vi "Initialize Battle Dialog.vi"() -> (1 "# Players":i32, 2 "Dashboard":T1[](array[typedef]), 3 "SquareBattle out":refnum<class "SquareBattle.lvclass">, 4 "Intensity Graph Values":cluster{dbl, u32}[](array[cluster]), 6 "Continue?":bool)   [LabVIEW 2014, in "SquareBattle.lvclass"]
uses:
  SquareBattle.lvclass
  Dashboard.ctl
  Runner/Runner.lvclass
  Runner/Runner.lvclass/Runner.ctl
  Runner Cluster.ctl
  SquareBattle.lvclass/SquareBattle.ctl
  Endigit Library/Endigit.lvlib
panel:
  in  "Default Colors":u32[](array[colorbox])=[11163013, 4877194, 13936746, 10864227, 9567230, 16776960, 12868095, 16762130]
  in  "Background Color":u32(colorbox)
  in  "Players":cluster{"Player":u16, "Color":u32}[](array[cluster]) {"Player" items=["Sleepy Engineer"=2, "Sleepy Engineer"=3, "Sleepy Engineer"=4, "Sleepy Engineer"=5, "Shawn the Explorer"=6, "Robert"=8, "Shawn the Wanderer"=9]}
  in  "Cancel":bool
  in  "Start":bool
  in  "Board size":i32=150
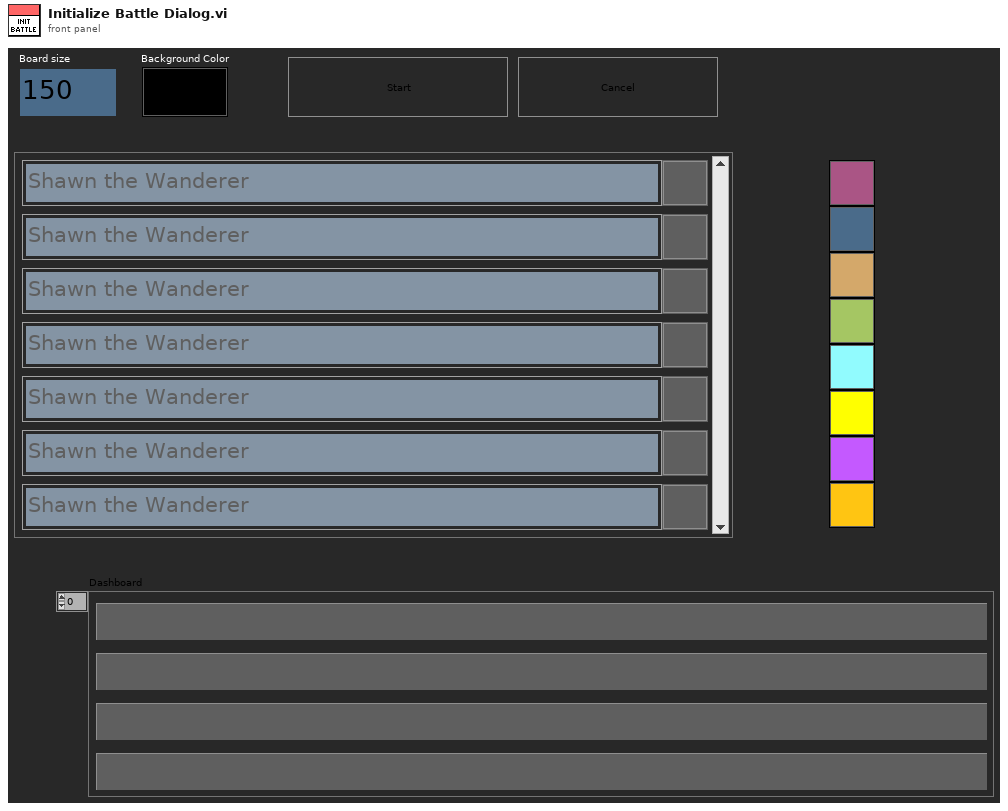
[diagram p1: front panel]
types:
  T1 = typedef "SquareBattle.lvclass/Dashboard.ctl" = cluster{"Color":u32, "Player":string, "Status":string}
  T2 = typedef "SquareBattle.lvclass/Player Info.ctl" = cluster{"Name":string, "Color Box":u32, "Gloat Phrase":string}
  T3 = typedef "SquareBattle.lvclass/Runner Cluster.ctl" = cluster{"Alive?":bool, "RunnerRef":refnum<data-value>, "TeamIdx":i32, "Player #":i32, "NextPlay":u32}
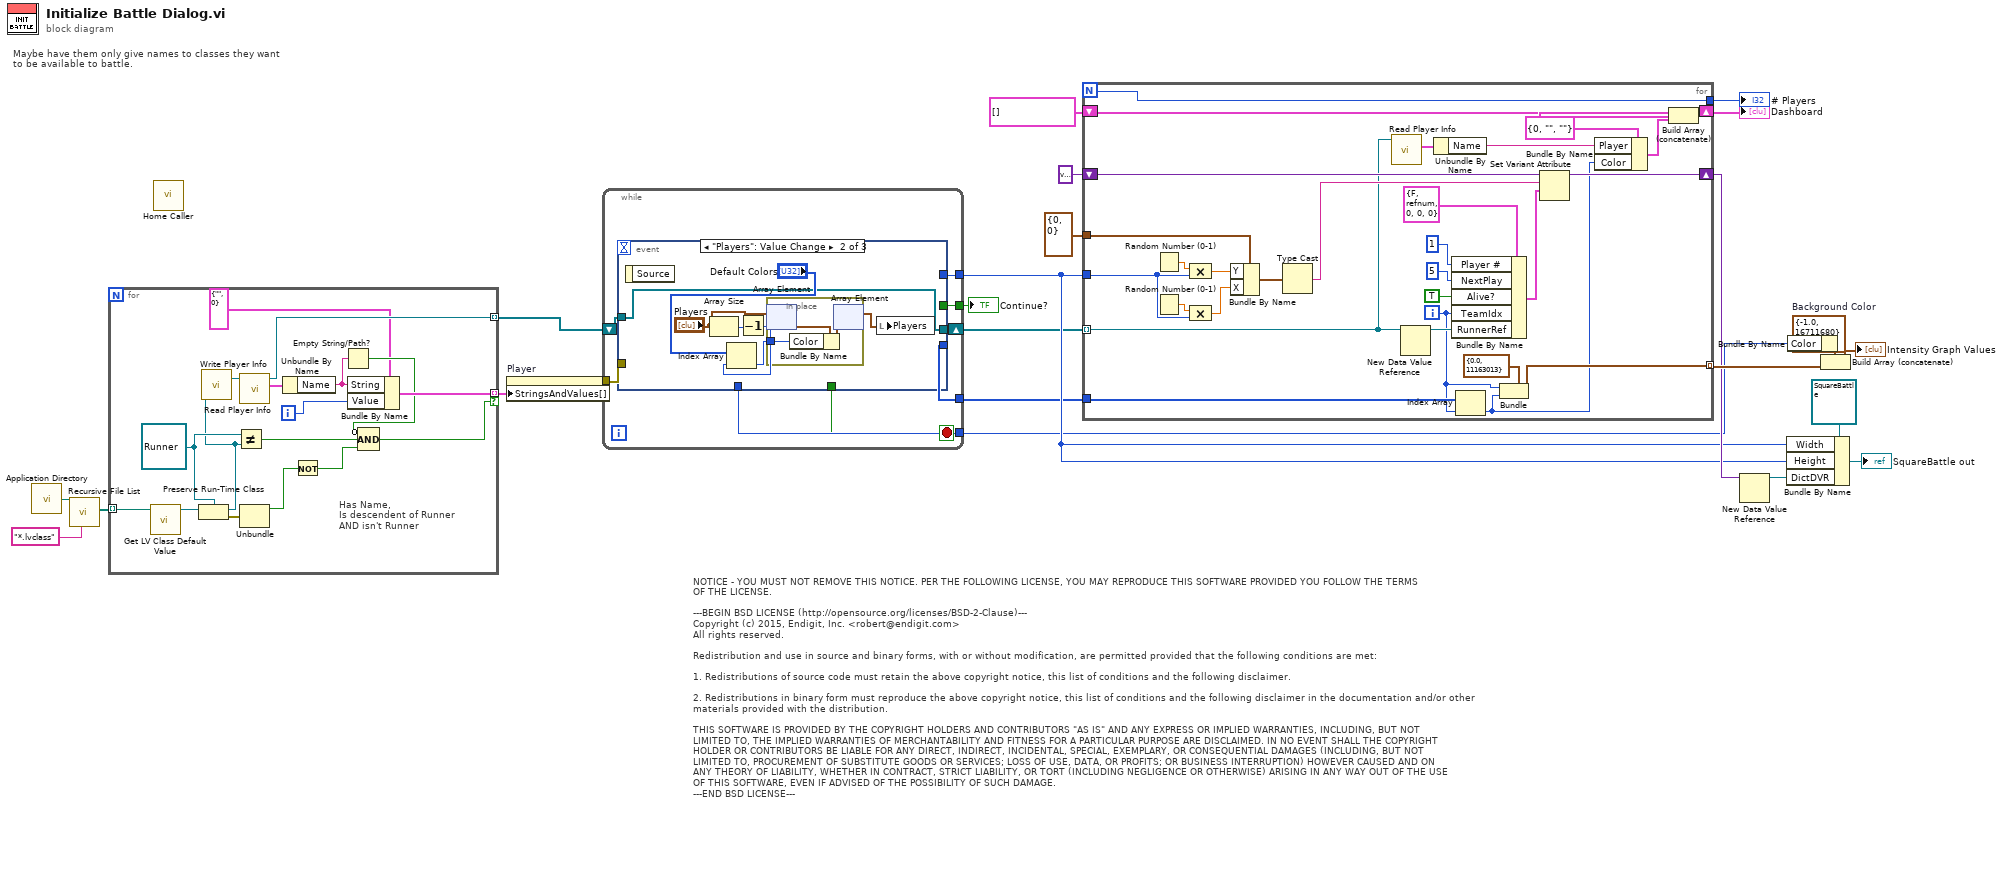
[diagram p0: block diagram]
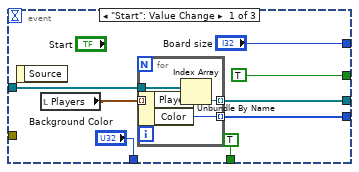
[diagram p2: hidden frame]
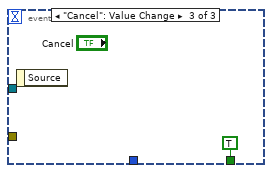
[diagram p3: hidden frame]
diagram:
  w11 = cluster{dbl, "Color":u32} {-1.0, "Color"=16711680}  # Background Color
  # "NOTICE - YOU MUST NOT REMOVE THIS NOTICE. PER THE FOLLOWING LICENSE, YOU MAY REPRODUCE THIS SOFTWARE PROVIDED YOU FOLLOW THE TERMS\nOF THE LICENSE.\n\n---BEGIN BSD LICENSE (http://opensource.org/licenses/BSD-2-Clause)---\nCopyright (c) 2015, Endigit, Inc. <robert@endigit.com>\nAll rights reserved.\n\nRedistribution and use in source and binary forms, with or without modification, are permitted provided that the following conditions are met:\n\n1. Redistributions of source code must retain the above copyright notice, this list of conditions and the following disclaimer.\n\n2. Redistributions in binary form must reproduce the above copyright notice, this list of conditions and the following disclaimer in the documentation and/or other \nmaterials provided with the distribution.\n\nTHIS SOFTWARE IS PROVIDED BY THE COPYRIGHT HOLDERS AND CONTRIBUTORS \"AS IS\" AND ANY EXPRESS OR IMPLIED WARRANTIES, INCLUDING, BUT NOT \nLIMITED TO, THE IMPLIED WARRANTIES OF MERCHANTABILITY AND FITNESS FOR A PARTICULAR PURPOSE ARE DISCLAIMED. IN NO EVENT SHALL THE COPYRIGHT \nHOLDER OR CONTRIBUTORS BE LIABLE FOR ANY DIRECT, INDIRECT, INCIDENTAL, SPECIAL, EXEMPLARY, OR CONSEQUENTIAL DAMAGES (INCLUDING, BUT NOT \nLIMITED TO, PROCUREMENT OF SUBSTITUTE GOODS OR SERVICES; LOSS OF USE, DATA, OR PROFITS; OR BUSINESS INTERRUPTION) HOWEVER CAUSED AND ON \nANY THEORY OF LIABILITY, WHETHER IN CONTRACT, STRICT LIABILITY, OR TORT (INCLUDING NEGLIGENCE OR OTHERWISE) ARISING IN ANY WAY OUT OF THE USE \nOF THIS SOFTWARE, EVEN IF ADVISED OF THE POSSIBILITY OF SUCH DAMAGE.\n---END BSD LICENSE---"
  # "Maybe have them only give names to classes they want \nto be available to battle."
  n1 = call <vilib>:"Application Directory.vi"() -> ("Application Directory"=w10:path)
  n2 = call <vilib>:"Recursive File List.vi"("pattern"="*.lvclass", "Folder Path"=w10) -> ("All Files in Dir"=w8:path[])  [unwired: 5 in, 4 out]
  n3 = for {
    tunnel: w8 -> [w41] mode=indexing
    tunnel: [w33] -> w2 mode=indexing if=w34
    tunnel: [w31] -> w7 mode=indexing
    i -> [w25]
    w36 = refnum<class "Runner.lvclass"> refnum ("Runner.lvclass")
    # "Has Name,\nIs descendent of Runner\nAND isn't Runner"
    n4 = call <vilib>:"Get LV Class Default Value.vi"("class path"=w41) -> ("object"=w40:refnum<class>)  [unwired: 9 in, 1 out]
    n5 = Preserve Run-Time Class(object in=w40, 2:w36) -> (object out=w32:refnum<class "Runner.lvclass">, error out=w39:errorcluster)  [unwired: 1 in]
    n6 = call-dynamic "Write Player Info.vi"("Runner in"=w32) -> ("Runner out"=w29:refnum<class "Runner.lvclass">)  [unwired: 9 in, 1 out]
    n7 = Not Equal?(x=w36, y=w32) -> (x != y?=w35:bool)
    n8 = call "Read Player Info.vi"("Runner in"=w29) -> ("Player Info"=w30:T2, "Runner out"=w31:refnum<class "Runner.lvclass">)  [unwired: 8 in, 1 out]
    n9 = Unbundle(w39) -> ("status"=w38:bool)  [unwired: 2 out]
    n10 = Unbundle By Name(w30) -> ("Name"=w28:string)
    n11 = Not(x=w38) -> (.not. x?=w37:bool)
    n12 = Empty String/Path?(string/path=w28) -> (empty?=w27:bool)
    n13 = Bundle By Name(cluster=cluster{"String":string, "Value":u16} {"String"="", "Value"=0}, "String"=w28, "Value"=w25) -> (w33:cluster{"String":string, "Value":u16})
    n14 = Compound Arithmetic op=AND(invert w27, w35, w37) -> (w34:bool)
  }
  n15 = call "Home Caller.vi"() -> ()  [unwired: 11 in]
  n16 = property on="Player" class="Ring (strict)"("StringsAndValues[]"=w2) -> (error out=w1:errorcluster)  [unwired: 2 in, 1 out]
  n17 = while {
    tunnel: [w49] -> w14
    tunnel: [w48] -> w13
    tunnel: [w45] -> w4
    tunnel: [w44] -> w3
    tunnel: w1 -> [w43]
    shift-right: [w46] -> w6
    shift-left: w7 -> [w47]
    stop <- w42 stop-if-true
    n18 = event shown="[1] \"Players\": Value Change" {
      selector: _ -> [_ _ _]
      dyn-events: _ -> [_ _ _]
      timeout: _ -> [_ _ _]
      tunnel: ["Board size" _ _] -> w49
      tunnel: [TRUE ("Start") _ _] -> w48
      tunnel: w47 -> [w55 w63 _]
      tunnel: [w54 w63 _] -> w46
      tunnel: ["Background Color" _ _] -> w45
      tunnel: [w51 _ _] -> w44
      tunnel: w43 -> [_ _ _]
      tunnel: [TRUE _ TRUE] -> w42
      event "Start": Value Change {
        n19 = event-data() -> ()  [unwired: 1 in, 1 out]
        n20 = local read "Players"() -> (w52:cluster{"Player":u16, "Color":u32}[])
        n21 = for {
          tunnel: w52 -> [w61] mode=indexing
          tunnel: w55 -> [w62]
          tunnel: [w60] -> w54 mode=indexing
          tunnel: [w58] -> w51 mode=indexing
          n22 = Unbundle By Name(w61) -> ("Player"=w59:u16, "Color"=w58:u32)
          n23 = Index Array(array=w62, index=w59) -> (element=w60:refnum<class "Runner.lvclass">)
        }
      }
      event "Players": Value Change {
        n24 = event-data() -> ()  [unwired: 1 in, 1 out]
        n25 = Array Size(array="Players") -> (size(s)=w69:i32)
        n26 = Decrement(x=w69) -> (x-1=w66:i32)
        n27 = Index Array(array="Default Colors", index=w66) -> (element=w65:u32)
        n28 = in-place {
          in-place-border: w65 -> [w70]
          n29 = in-place-array #1("Players", w66) -> (w72:cluster{"Player":u16, "Color":u32})
          n30 = Bundle By Name(cluster=w72, "Color"=w70) -> (w71:cluster{"Player":u16, "Color":u32})
          n31 = in-place-array #1(w71) -> (w64:cluster{"Player":u16, "Color":u32}[])  [unwired: 1 out]
        }
        n32 = local write "Players"(w64) -> ()
      }
      event "Cancel": Value Change {
        n33 = event-data() -> ()  [unwired: 1 in, 1 out]
      }
    }
  }
  "Continue?" <- w13
  n34 = for {
    N -> [w82]
    tunnel: w6 -> [w74] mode=indexing
    shift-right: [w96] -> w19
    shift-left: variant -> [w100]
    tunnel: cluster{"Y":i32, "X":i32} {"Y"=0, "X"=0} -> [w99]
    shift-right: [w90] -> w23
    shift-left: T1[] [] ("Dashboard") -> [w89]
    tunnel: [w78] -> w22 mode=indexing
    tunnel: w14 -> [w84]
    tunnel: [w82] -> w24
    tunnel: w3 -> [w77]
    i -> [w75]
    n35 = Random Number (0-1)() -> (number: 0 to 1=w87:dbl)
    n36 = Random Number (0-1)() -> (number: 0 to 1=w85:dbl)
    n37 = Compound Arithmetic op=MULTIPLY(w87, w84) -> (w86:dbl)
    n38 = Compound Arithmetic op=MULTIPLY(w85, w84) -> (w83:dbl)
    n39 = Bundle By Name(cluster=w99, "Y"=w86, "X"=w83) -> (w98:cluster{"Y":i32, "X":i32})
    n40 = Type Cast(x=w98) -> (*(type *) &x=w97:string)  [unwired: 1 in]
    n41 = call "Read Player Info.vi"("Runner in"=w74) -> ("Player Info"=w81:T2)  [unwired: 8 in, 2 out]
    n42 = New Data Value Reference(data value=w74) -> (data value reference=w93:refnum<data-value>)  [unwired: 1 in, 1 out]
    n43 = Unbundle By Name(w81) -> ("Name"=w80:string)
    n44 = Bundle By Name(cluster=T3 {"Alive?"=FALSE, "RunnerRef"=refnum, "TeamIdx"=0, "Player #"=0, "NextPlay"=0} ("Cluster"), "Player #"=1, "NextPlay"=u32 5 ("Y Loc"), "Alive?"=TRUE, "TeamIdx"=w75, "RunnerRef"=w93) -> (w92:T3)
    n45 = Index Array(array=w77, index=w75) -> (element=w76:u32)
    n46 = Bundle(cluster=cluster{dbl, u32} {0.0, 11163013}, w75, w76) -> (w78:cluster{dbl, u32})
    n47 = Set Variant Attribute(Variant=w100, name=w97, value=w92) -> (Variant out=w96:variant)  [unwired: 1 in, 2 out]
    n48 = Bundle By Name(cluster=T1 {"Color"=0, "Player"="", "Status"=""} ("Dashboard"), "Player"=w80, "Color"=w76) -> (w88:T1)
    n49 = Build Array (concatenate)(w89, w88) -> (w90:T1[])
  }
  "# Players" <- w24
  "Dashboard" <- w23
  n50 = New Data Value Reference(data value=w19) -> (data value reference=w16:refnum<data-value>)  [unwired: 1 in, 1 out]
  n51 = Bundle By Name(cluster=refnum<class "SquareBattle.lvclass"> refnum ("Maze 2.0.lvclass"), "Width"=w14, "Height"=w14, "DictDVR"=w16) -> (→"SquareBattle out":refnum<class "SquareBattle.lvclass">)
  n52 = Bundle By Name(cluster=w11, "Color"=w4) -> (w5:cluster{dbl, "Color":u32})
  n53 = Build Array (concatenate)(w5, w22) -> (→"Intensity Graph Values":cluster{dbl, "Color":u32}[])
